vi "命令记录.vi"(10 "填充元素":string, 11 "填充数组":string[](array[string])) -> (2 "已处理命令":string, 3 "填充数组输出":string[](array[string]))   [LabVIEW 2016]
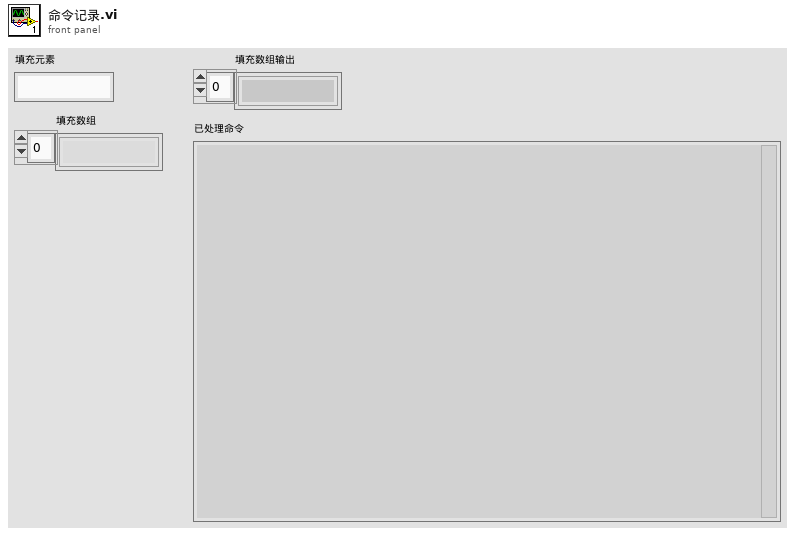
[diagram p1: front panel]
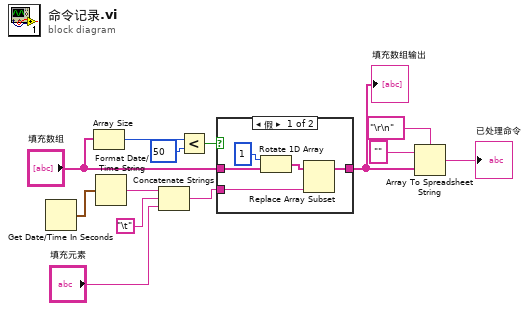
[diagram p0: block diagram]
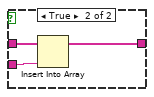
[diagram p2: hidden frame]
diagram:
  n1 = Get Date/Time In Seconds() -> (seconds since 1Jan1904=w1:timestamp)
  n2 = Array Size(array="填充数组") -> (size(s)=w10:i32)
  n3 = Format Date/Time String(seconds (now)=w1) -> (date/time string=w2:string)  [unwired: 2 in]
  n4 = Concatenate Strings(w2, "\t", "填充元素") -> (w7:string)
  n5 = Less?(x=w10, y=50) -> (x < y?=w12:bool)
  n6 = case shown="假" w12 {
    tunnel: w7 -> [w15 w20]
    tunnel: "填充数组" -> [w17 w21]
    tunnel: [w14 w19] -> w13
    frame False {
      n7 = Rotate 1D Array(1:w17, 2:1 ("n")) -> (0:w16:string[])
      n8 = Replace Array Subset(array=w16, new element=w15) -> (w14:string[])  [unwired: 1 in]
    }
    frame True {
      n9 = Insert Into Array(array=w21, new element=w20) -> (w19:string[])  [unwired: 1 in]
    }
  }
  "填充数组输出" <- w13
  n10 = Array To Spreadsheet String(delimiter (Tab)="\r\n" ("分隔符(Tab)"), array=w13, 3:"" ("格式字符串")) -> (spreadsheet string=→"已处理命令":string)
